vi "Aero_tunnel_monitor_orig.vi"(1 "path in":path=path "C:/Aerotech/Drivers/OGI_IF.dll") -> ()   [LabVIEW 2010]
uses:
  ADAM Client/Sub VIs/ADAM Controls/Update_scan_value.ctl
  Aero_Tunnel_Server_Global.vi
panel:
  out "SmAD Data":dbl[](array[numeric]) format="%.2f"
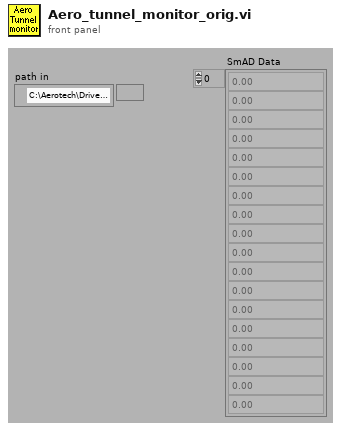
[diagram p1: front panel]
types:
  T1 = typedef "Update_scan_value.ctl" = cluster{"Channel Name":string, "New Value":dbl}
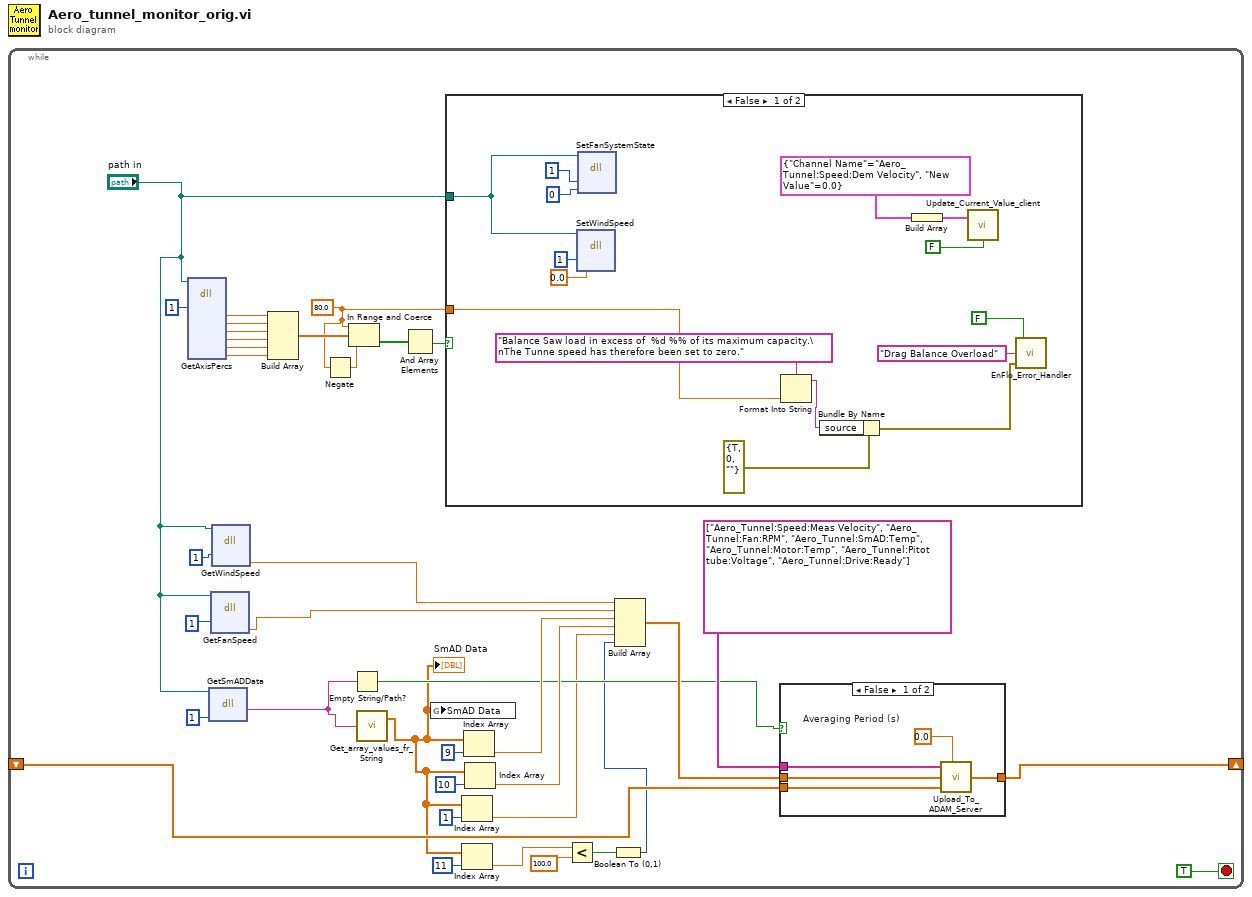
[diagram p0: block diagram]
diagram:
  n1 = while {
    shift-right: [w16] -> _
    shift-left: _ -> [w12]
    stop <- TRUE stop-if-true
    w26 = 80.0 ("upper limit")
    n2 = dll-call lib="C:/Aerotech/Drivers/OGI_IF.dll" fn="GetAxisPercs"(path in="path in", "Enable"=1) -> ("Lift"=w36:dbl, "Pitch"=w35:dbl, "Drag"=w34:dbl, "side"=w33:dbl, "Yaw"=w32:dbl, "Roll"=w31:dbl)  [unwired: 3 in, 9 out]
    n3 = dll-call lib="C:/Aerotech/Drivers/OGI_IF.dll" fn="GetSmADData"(path in="path in", "Enable"=1) -> ("SmAD Data String"=w17:string)  [unwired: 3 in, 2 out]
    n4 = dll-call lib="C:/Aerotech/Drivers/OGI_IF.dll" fn="GetFanSpeed"(path in="path in", "Enable"=1) -> ("FanSpeedinRPM"=w22:dbl)  [unwired: 3 in, 4 out]
    n5 = dll-call lib="C:/Aerotech/Drivers/OGI_IF.dll" fn="GetWindSpeed"(path in="path in", "Enable"=1) -> ("Windspeed_M/s"=w23:dbl)  [unwired: 3 in, 4 out]
    n6 = Build Array(w36, w35, w34, w33, w32, w31) -> (w30:dbl[])
    n7 = Negate(x=w26) -> (-x=w27:dbl)
    n8 = In Range and Coerce(upper limit=w26, x=w30, lower limit=w27) -> (In Range?=w29:bool[])  [unwired: 1 out]
    n9 = Empty String/Path?(string/path=w17) -> (empty?=w9:bool)
    n10 = call "Get_array_values_fr_String.vi"("String Value"=w17) -> ("Numeric Array"=w5:dbl[])  [unwired: 1 out]
    "SmAD Data" <- w5
    n11 = And Array Elements(Boolean array=w29) -> (logical AND=w28:bool)
    n12 = global write "Aero_Tunnel_Server_Global.vi" "SmAD Data"(w5) -> ()
    n13 = case shown="False" w28 {
      tunnel: "path in" -> [w47 _]
      tunnel: w26 -> [w56 _]
      frame False {
        n14 = dll-call lib="C:/Aerotech/Drivers/OGI_IF.dll" fn="SetWindSpeed"(path in=w47, "Enable"=1, "NewWindSpeed"=0.0) -> ()  [unwired: 4 in, 3 out]
        n15 = dll-call lib="C:/Aerotech/Drivers/OGI_IF.dll" fn="SetFanSystemState"(path in=w47, "Enable"=1, "Fan ONOFF"=0) -> ()  [unwired: 4 in, 3 out]
        n16 = Format Into String(format string="Balance Saw load in excess of  %d %% of its maximum capacity.\nThe Tunne speed has therefore been set to zero.", w56) -> (resulting string=w53:string)  [unwired: 2 in, 1 out]
        n17 = Bundle By Name(cluster=errorcluster {"status"=TRUE, "code"=0, "source"=""} ("error in (no error)"), "source"=w53) -> (w52:errorcluster)
        n18 = Build Array(T1 {"Channel Name"="Aero_Tunnel:Speed:Dem Velocity", "New Value"=0.0} ("Update Scan Value Cluster")) -> (w45:T1[])
        n19 = call "Update_Current_Value_client.vi"("Don't Bother with check?"=FALSE, "Update array in"=w45) -> ()
        n20 = call "EnFlo_Error_Handler.vi"("error in (no error)"=w52, "Error Type"="Drag Balance Overload", "Dialog Box (T)"=FALSE) -> ()  [unwired: 3 out]
      }
      frame True {
      }
    }
    n21 = Index Array(array=w5, index=1) -> (element=w7:dbl)
    n22 = Index Array(array=w5, index=11) -> (element=w4:dbl)
    n23 = Index Array(array=w5, index=9) -> (element=w15:dbl)
    n24 = Index Array(array=w5, index=10) -> (element=w14:dbl)
    n25 = Less?(x=w4, y=100.0) -> (x < y?=w2:bool)
    n26 = Boolean To (0,1)(Boolean=w2) -> (0, 1=w1:i16)
    n27 = Build Array(w23, w22, w15, w14, w7, w1) -> (w13:dbl[])
    n28 = case shown="False" w9 {
      tunnel: [w42 w43] -> w16
      tunnel: w12 -> [w41 w43]
      tunnel: string[] ["Aero_Tunnel:Speed:Meas Velocity", "Aero_Tunnel:Fan:RPM", "Aero_Tunnel:SmAD:Temp", "Aero_Tunnel:Motor:Temp", "Aero_Tunnel:Pitot tube:Voltage", "Aero_Tunnel:Drive:Ready"] ("Channel Names") -> [w40 _]
      tunnel: w13 -> [w39 _]
      frame False {
        w38 = 0.0  # Averaging Period (s)
        n29 = call "Upload_To_ADAM_Server.vi"("Channel Names"=w40, "Averaging Period (s)"=w38, "Channel Values"=w39, "Shift In"=w41) -> ("Shift Out"=w42:dbl[])  [unwired: 1 out]
      }
      frame True {
      }
    }
  }
